vi "Test-Host-AES-Single-Round.vi"() -> ()   [LabVIEW 2017]
panel:
  out "_a (U32)":u32[](array[numeric]) format="%.0x"
  out "Pass?":bool
  out "exp_c":u32[](array[numeric]) format="%.0x"
  out "act_c":u32[](array[numeric]) format="%.0x"
  out "_c":u32[](array[numeric]) format="%.0x"
  out "_a":u64[](array[numeric]) format="%.0x"
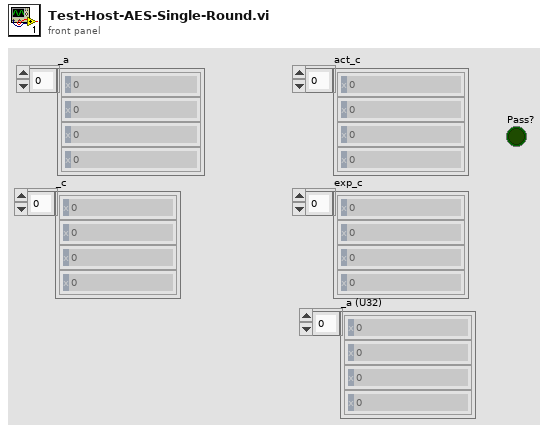
[diagram p1: front panel]
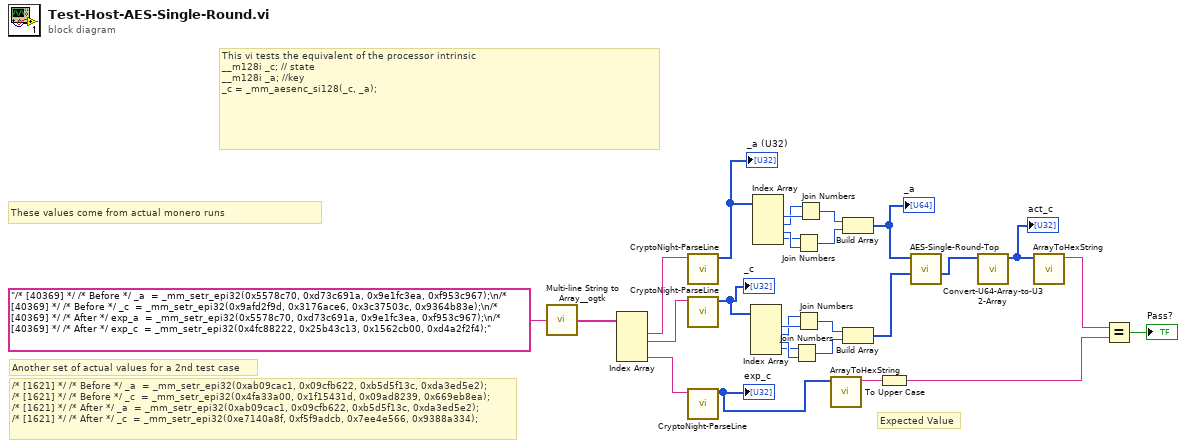
[diagram p0: block diagram]
diagram:
  # "Another set of actual values for a 2nd test case"
  # "/* [1621] */ /* Before */ _a  = _mm_setr_epi32(0xab09cac1, 0x09cfb622, 0xb5d5f13c, 0xda3ed5e2);\n/* [1621] */ /* Before */ _c  = _mm_setr_epi32(0x4fa33a00, 0x1f15431d, 0x09ad8239, 0x669eb8ea);\n/* [1621] */ /* After */ _a  = _mm_setr_epi32(0xab09cac1, 0x09cfb622, 0xb5d5f13c, 0xda3ed5e2);\n/* [1621] */ /* After */ _c  = _mm_setr_epi32(0xe7140a8f, 0xf5f9adcb, 0x7ee4e566, 0x9388a334);"
  # "Expected Value"
  # "This vi tests the equivalent of the processor intrinsic\n__m128i _c; // state\n__m128i _a; //key\n_c = _mm_aesenc_si128(_c, _a);"
  # "These values come from actual monero runs"
  n1 = call <userlib>:"Multi-line String to Array__ogtk.vi"("string"="/* [40369] */ /* Before */ _a  = _mm_setr_epi32(0x5578c70, 0xd73c691a, 0x9e1fc3ea, 0xf953c967);\n/* [40369] */ /* Before */ _c  = _mm_setr_epi32(0x9afd2f9d, 0x3176ace6, 0x3c37503c, 0x9364b83e);\n/* [40369] */ /* After */ exp_a  = _mm_setr_epi32(0x5578c70, 0xd73c691a, 0x9e1fc3ea, 0xf953c967);\n/* [40369] */ /* After */ exp_c  = _mm_setr_epi32(0x4fc88222, 0x25b43c13, 0x1562cb00, 0xd4a2f2f4);") -> ("lines"=w25:string[])
  n2 = Index Array(array=w25) -> (element #1=w28:string, element #2=w27:string, element #4=w26:string)  [unwired: 4 in, 1 out]
  n3 = call "CryptoNight-ParseLine.vi"("line"=w28) -> ("Array"=w11:u32[])  [unwired: 10 in]
  "_a (U32)" <- w11
  n4 = call "CryptoNight-ParseLine.vi"("line"=w27) -> ("Array"=w4:u32[])  [unwired: 10 in]
  "_c" <- w4
  n5 = call "CryptoNight-ParseLine.vi"("line"=w26) -> ("Array"=w22:u32[])  [unwired: 10 in]
  "exp_c" <- w22
  n6 = Index Array(array=w4) -> (element #1=w10:u32, element #2=w9:u32, element #3=w8:u32, element #4=w7:u32)  [unwired: 4 in]
  n7 = Index Array(array=w11) -> (element #1=w18:u32, element #2=w17:u32, element #3=w16:u32, element #4=w15:u32)  [unwired: 4 in]
  n8 = Join Numbers(hi=w7, lo=w8) -> ((hi.lo)=w6:u64)
  n9 = Join Numbers(hi=w15, lo=w16) -> ((hi.lo)=w14:u64)
  n10 = Join Numbers(hi=w9, lo=w10) -> ((hi.lo)=w5:u64)
  n11 = Join Numbers(hi=w17, lo=w18) -> ((hi.lo)=w13:u64)
  n12 = call "ArrayToHexString.vi"("U32 Array"=w22) -> ("String"=w21:string)  [unwired: 10 in]
  n13 = Build Array(w13, w14) -> (w12:u64[])
  "_a" <- w12
  n14 = Build Array(w5, w6) -> (w3:u64[])
  n15 = To Upper Case(1:w21) -> (0:w23:string)
  n16 = call "AES-Single-Round-Top.vi"("state (_c) U64"=w3, "key (_a)"=w12) -> ("state out (c) U64"=w2:u64[])  [unwired: 9 in]
  n17 = call "Convert-U64-Array-to-U32-Array.vi"("2 x U64"=w2) -> ("4 x U32"=w1:u32[])  [unwired: 10 in]
  "act_c" <- w1
  n18 = call "ArrayToHexString.vi"("U32 Array"=w1) -> ("String"=w20:string)  [unwired: 10 in]
  n19 = Equal?(x=w20, y=w23) -> (x = y?=→"Pass?":bool)
